vi "servoPos (SubVI).vi"(7 "Servos":T1, 8 "error in (no error)":errorcluster, 10 "ServoPosition (us)":dbl(slide)=1500.0 scale=500.0..2500.0, 11 "ServosRef in":refnum<class "PWM Generator.lvclass">[](array[class])) -> (0 "error out":errorcluster, 3 "ServosRef out":refnum<class "PWM Generator.lvclass">[](array[class]))   [LabVIEW 2020]
uses:
  <vilib>/CISH Robotics/L4VMX VMXpi/PWM Generator/PWM Generator.lvclass
  servoName.ctl
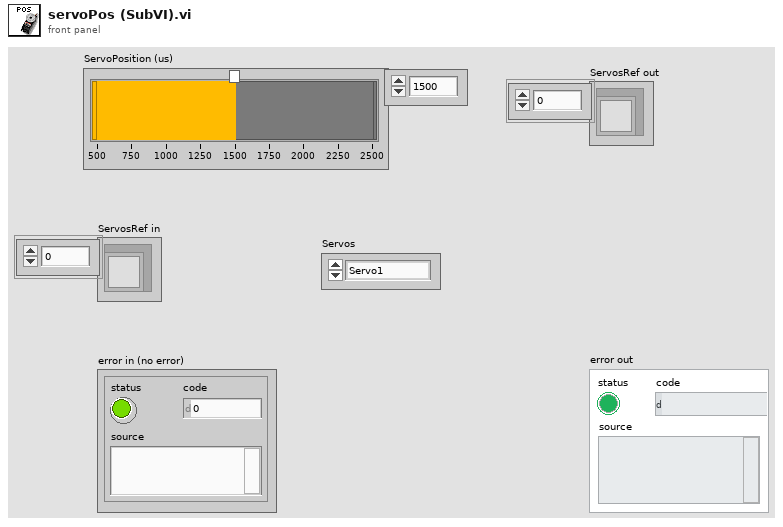
[diagram p1: front panel]
types:
  T1 = typedef "servoName.ctl" = enum16{"Servo1", "Servo2", "Servo3", "Servo4"}
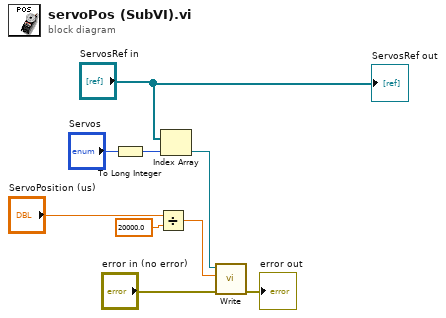
[diagram p0: block diagram]
diagram:
  n1 = To Long Integer(number="Servos") -> (32bit integer=w1:i32)
  n2 = Divide(x="ServoPosition (us)", y=20000.0) -> (x/y=w5:dbl)
  n3 = Index Array(array="ServosRef in", index=w1) -> (element=w6:refnum<class "PWM Generator.lvclass">)
  n4 = call <vilib>:"Write.vi"("Error In"="error in (no error)", "Duty Cycle(0~1)"=w5, "PWM Generator Object"=w6) -> ("Error Out"=→"error out":errorcluster)  [unwired: 7 in, 1 out]
  "ServosRef out" <- "ServosRef in"
